vi "IPS Ctrl Persistent Heater.vi"(3 "Error In":errorcluster={"status"=FALSE, "code"=1073676294, "source"="VISA Read in Prologix USB GPIB Command.vi"}, 4 "Activity":i32(listbox)=1, 5 "VISA resource name (COM Port of Prologix Device)":refnum<visa-resource-name>="GPIB0::24::INSTR") -> (0 "Error Out":errorcluster={"status"=FALSE, "code"=1073676293, "source"="VISA Read in NI USB GPIB Command.vi->IPS Ctrl Persistent Heater.vi"}, 2 "Output":string="H\r")   [LabVIEW 2016]
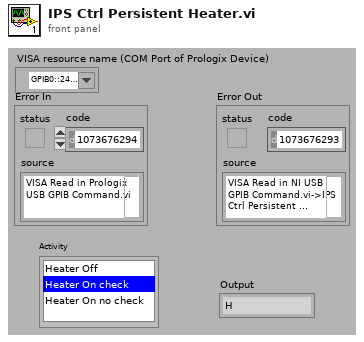
[diagram p1: front panel]
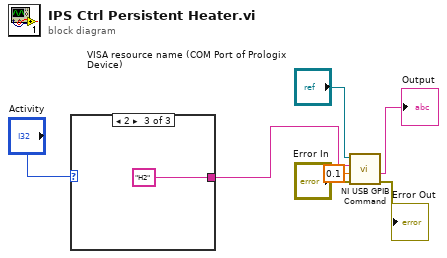
[diagram p0: block diagram]
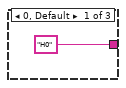
[diagram p2: hidden frame]
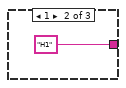
[diagram p3: hidden frame]
diagram:
  n1 = case shown="2" "Activity" {
    tunnel: ["H0" "H1" "H2"] -> w1
    frame 0, Default {
    }
    frame 1 {
    }
    frame 2 {
    }
  }
  n2 = call "NI USB GPIB Command.vi"("Error In"="Error In", "Wait for instrument to respond (s)"=0.1, "String to Send"=w1, "VISA resource name (COM Port of Prologix Device)"="VISA resource name (COM Port of Prologix Device)") -> ("Error Out"=→"Error Out":errorcluster, "Return String from Device (Not all commands return a String)"=→"Output":string)  [unwired: 2 out]
